vi "Init_Cluster_Various_Things-1.vi"() -> (0 "Test cluster":T1)   [LabVIEW 2013]
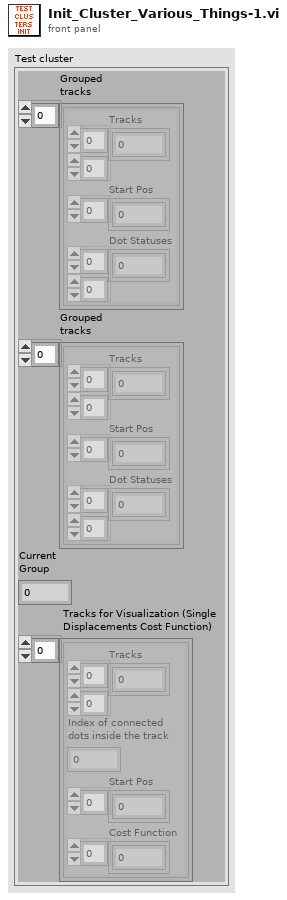
[diagram p1: front panel]
types:
  T1 = cluster{"Grouped \ntracks":cluster{"Tracks":dbl[][], "Start Pos":i32[], "Dot Statuses":i16[][]}[], "Grouped \ntracks":cluster{"Tracks":dbl[][], "Start Pos":i32[], "Dot Statuses":i16[][]}[], "Current\nGroup":i32, " Tracks for Visualization (Single\n Displacements Cost Function)":cluster{"Tracks":dbl[][], "Index of connected \ndots inside the track":i32, "Start Pos":i32[], "Cost Function":u8[]}[]}
  T2 = cluster{"Tracks":dbl[][], "Index of connected \ndots inside the track":i32, "Start Pos":i32[], "Cost Function":u8[]}[]
  T3 = cluster{"Tracks":dbl[][], "Start Pos":i32[], "Dot Statuses":i16[][]}[]
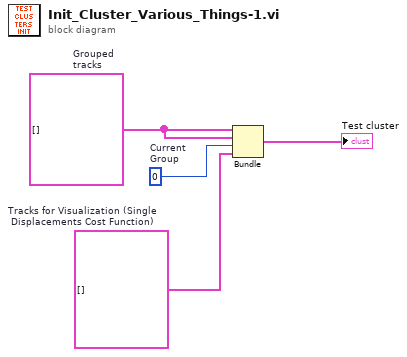
[diagram p0: block diagram]
diagram:
  w2 = T2 []  # Tracks for Visualization (Single  Displacements Cost Function)
  w3 = T3 []  # Grouped  tracks
  w4 = 0  # Current Group
  n1 = Bundle("Grouped \ntracks"=w3, "Grouped \ntracks"=w3, "Current\nGroup"=w4, "Tracks for Visualization (Single\n Displacements Cost Function)"=w2) -> (→"Test cluster":T1)  [unwired: 1 in]
